vi "lights_relay_data.vi"(4 "C2":bool, 5 "A1":bool, 6 "C1":bool, 7 "A2":bool, 8 "mode":T7, 9 "B2":bool, 10 "B1":bool, 11 "relays":T6) -> ()   [LabVIEW 2011]
uses:
  lights_led_mode.ctl
  <vilib>/Rock Robotics/WPI/Relay/WPI_RelayDevRef.ctl
  <vilib>/Rock Robotics/SystemInterfaces/DIO/FPGA_DIORelayChannel.ctl
  <vilib>/Rock Robotics/SystemInterfaces/Typedef/FPGA_TypedefDigitalModule.ctl
  <vilib>/Rock Robotics/WPI/Relay/WPI_RelayDirection.ctl
  <vilib>/Rock Robotics/WPI/Relay/WPI_RelayValue.ctl
panel:
  in  "digital truth table":T1[][](array[typedef])=[[enum."Off", enum."Forward"], [enum."Reverse", enum."On"]]
  in  "mode truth table":T1[](array[typedef])=[enum."Forward", enum."Reverse", enum."On"]
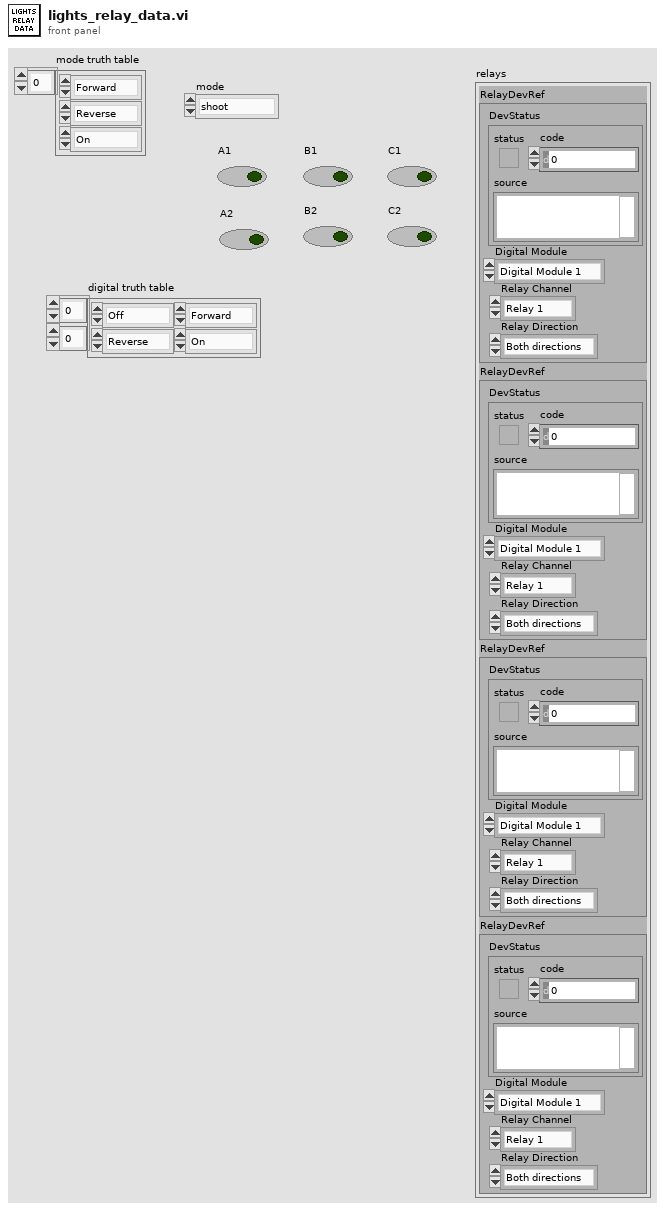
[diagram p1: front panel]
types:
  T1 = typedef "WPI_RelayValue.ctl" = enum16{"Off", "On", "Forward", "Reverse"}
  T2 = typedef "WPI_RelayDevRef.ctl" = cluster{"DevStatus":errorcluster, "Relay Channel":T3, "Digital Module":T4, "Relay Direction":T5}
  T3 = typedef "FPGA_DIORelayChannel.ctl" = enum8{"Relay 1", "Relay 2", "Relay 3", "Relay 4", "Relay 5", "Relay 6", "Relay 7", "Relay 8", "Invalid"}
  T4 = typedef "FPGA_TypedefDigitalModule.ctl" = enum16{"Digital Module 1", "Digital Module 2"}
  T5 = typedef "WPI_RelayDirection.ctl" = enum16{"Both directions", "Forward only", "Reverse only"}
  T6 = cluster{"RelayDevRef":T2, "RelayDevRef":T2, "RelayDevRef":T2, "RelayDevRef":T2}
  T7 = typedef "lights_led_mode.ctl" = enum16{"shoot", "balance", "indicator"}
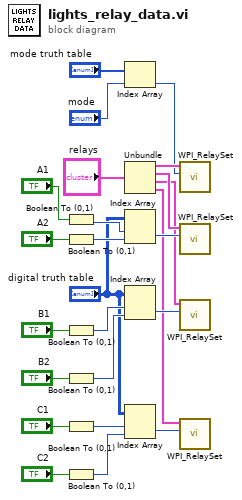
[diagram p0: block diagram]
diagram:
  n1 = Boolean To (0,1)(Boolean="A1") -> (0, 1=w16:i16)
  n2 = Boolean To (0,1)(Boolean="A2") -> (0, 1=w15:i16)
  n3 = Boolean To (0,1)(Boolean="B1") -> (0, 1=w12:i16)
  n4 = Boolean To (0,1)(Boolean="B2") -> (0, 1=w11:i16)
  n5 = Boolean To (0,1)(Boolean="C1") -> (0, 1=w9:i16)
  n6 = Boolean To (0,1)(Boolean="C2") -> (0, 1=w8:i16)
  n7 = Index Array(array="mode truth table", index="mode") -> (element=w20:T1)
  n8 = Unbundle("relays") -> ("RelayDevRef"=w23:T2, "RelayDevRef"=w18:T2, "RelayDevRef"=w6:T2, "RelayDevRef"=w5:T2)
  n9 = Index Array(array="digital truth table", index (row)=w16, index (col)=w15) -> (element=w19:T1)
  n10 = Index Array(array="digital truth table", index (row)=w12, index (col)=w11) -> (element=w13:T1)
  n11 = Index Array(array="digital truth table", index (row)=w9, index (col)=w8) -> (element=w10:T1)
  n12 = call <vilib>:"WPI_RelaySet.vi"("RelayValue"=w20, "RelayDevRef"=w23) -> ()  [unwired: 8 in, 2 out]
  n13 = call <vilib>:"WPI_RelaySet.vi"("RelayValue"=w19, "RelayDevRef"=w18) -> ()  [unwired: 8 in, 2 out]
  n14 = call <vilib>:"WPI_RelaySet.vi"("RelayValue"=w13, "RelayDevRef"=w6) -> ()  [unwired: 8 in, 2 out]
  n15 = call <vilib>:"WPI_RelaySet.vi"("RelayValue"=w10, "RelayDevRef"=w5) -> ()  [unwired: 8 in, 2 out]
